vi "MD5Checksum string.vi"(11 "Message String":string) -> (3 "MD5 message-digest":string)   [LabVIEW 2016]
doc: "This VI computes the MD5 message-digest of a string, based on the algorithm described in RFC 1321 (http://www.ietf.org/rfc/rfc1321.txt). The MD5 message-digest is a 128-bit number, displayed in lower case hexadecimal."
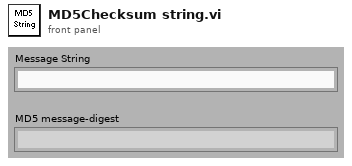
[diagram p1: front panel]
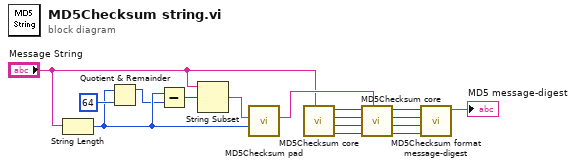
[diagram p0: block diagram]
diagram:
  n1 = String Length(string="Message String") -> (length=w4:i32)
  n2 = Quotient & Remainder(x=w4, y=64) -> (x-y*floor(x/y)=w3:i32)  [unwired: 1 out]
  n3 = Subtract(x=w4, y=w3) -> (x-y=w5:i32)
  n4 = String Subset(string="Message String", offset (0)=w5) -> (substring=w2:string)  [unwired: 1 in]
  n5 = call "MD5Checksum pad.vi"("Message String Length (bytes)"=w4, "Last Part of Message String"=w2) -> ("Padding"=w15:string)  [unwired: 9 in]
  n6 = call "MD5Checksum core.vi"("Input String"="Message String") -> ("s4 out"=w11:u32, "s3 out"=w12:u32, "s2 out"=w13:u32, "s1 out"=w14:u32)  [unwired: 7 in]
  n7 = call "MD5Checksum core.vi"("Input String"=w15, "s4 in"=w11, "s3 in"=w12, "s2 in"=w13, "s1 in"=w14) -> ("s4 out"=w7:u32, "s3 out"=w8:u32, "s2 out"=w9:u32, "s1 out"=w10:u32)  [unwired: 3 in]
  n8 = call "MD5Checksum format message-digest.vi"("s4"=w7, "s3"=w8, "s2"=w9, "s1"=w10) -> ("MD5 message-digest"=→"MD5 message-digest":string)  [unwired: 7 in]
